vi "Save-Recall Data.vi"(0 "VISA resource name":refnum<visa-resource-name>, 1 "data type (0 : raw data)":u16(ring) items=["raw data", "error-corrected data", "error-corrected trace memory", "formatted data", "formatted memory", "formatted data / memory", "formatted data - memory"], 3 "format (0:format 1)":u16(ring) items=["format 1 (6 byte internal)", "format 2 (8 byte IEEE 32 bit float)", "format 3 (16 byte IEEE 64 bit float)", "format 4 (50 byte ASCII)"], 4 "file name (read description)":path, 5 "error in (no error)":errorcluster, 6 "save/recall":bool, 7 "saver's name":string, 8 "saved data title":string, 9 "saved data comments":string) -> (12 "recaller's name":string, 14 "VISA resource name out":refnum<visa-resource-name>, 15 "recalled data title":string, 16 "recalled data comments":string, 17 "recalled data date":string, 18 "recalled data time":string, 19 "error out":errorcluster)   [LabVIEW 2018, in "Agilent 87XX Series.lvlib"]
doc: "This VI for the HP8753B Network Analyzer is used to save and recall data and memory traces and raw data.\n\n There are many differenent data arrays which can be read out of the instrument. If a 2-port calibration is active, the \"raw data\" consists of 4 arrays. Otherwise \"raw data\" as with the other data arrays, is just one array. Each type of data is saved into a single file. \"Raw data\" just requires a little more work to be decoded from the file and written back to the instrument. \n\n \"Trace memory\" can not be written back to the instrument as memory. It must be written back to the instrument as regular data which can then be rewritten to memory using the \"data to memory\" button or VI. This only works if the \"trace memory\" was the error-corrected memory and not the formatted memory. \n\n A few important notes...\n\n Recalling data seems to be a pretty temporary thing. For example, when data is recalled it is not overwriting the data that is already in the data arrays. The recalled data will be displayed, and it will be the data stored to memory, but changing the display causes the recalled to be lost and the old data to be displayed again.\n\n Whenever formatted data is saved, the display changes to reflect the data being saved. Example, saving \"formatted memory\" causes the display to switch to \"MEMORY\". Restoring data, switches the display to \"DATA\"."
uses:
  Agilent 87XX Series.lvlib
panel:
  # "save to file\nrecall from file"
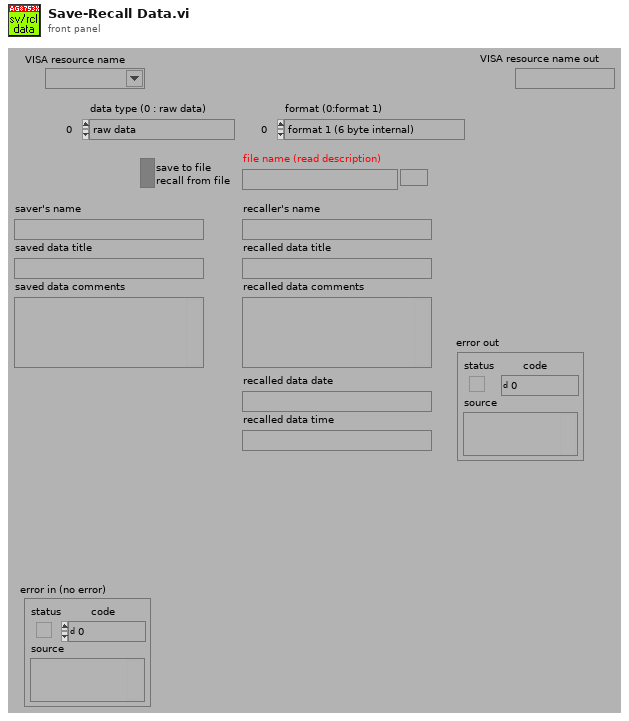
[diagram p1: front panel]
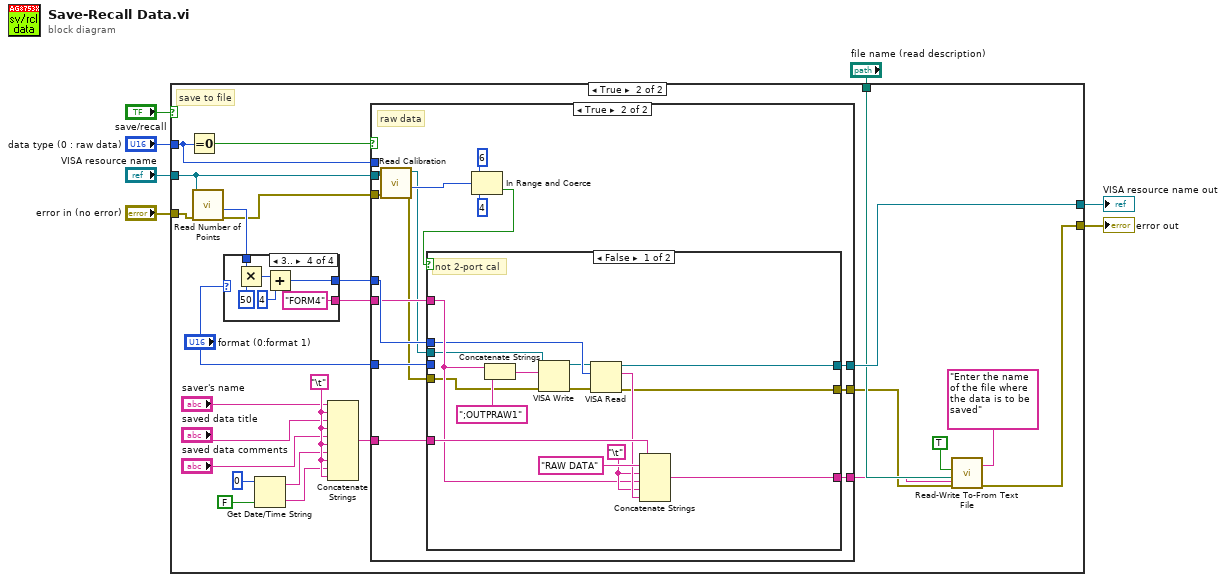
[diagram p0: block diagram]
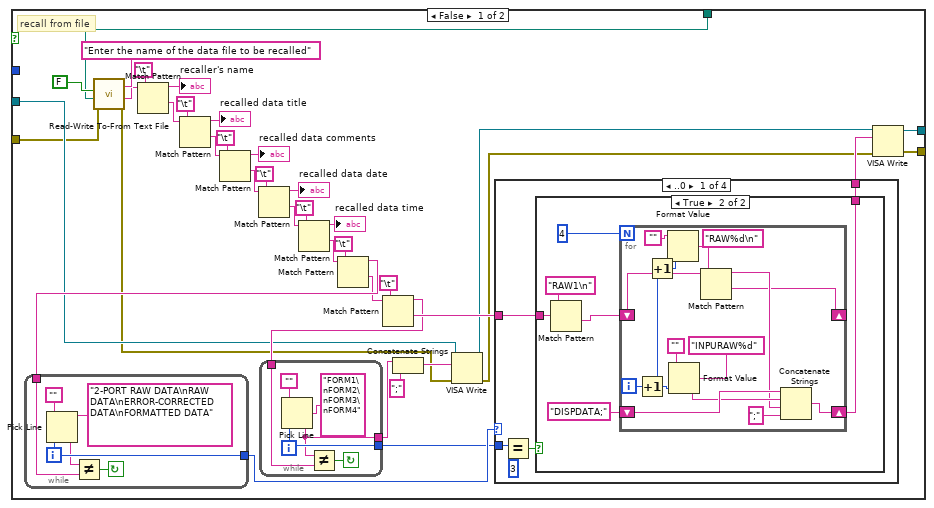
[diagram p2: hidden frame]
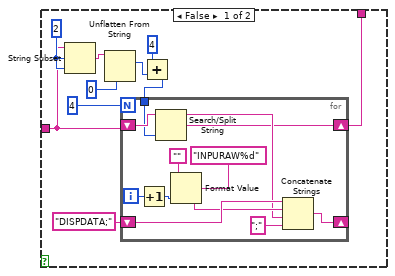
[diagram p3: hidden frame]
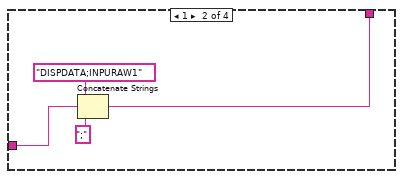
[diagram p4: hidden frame]
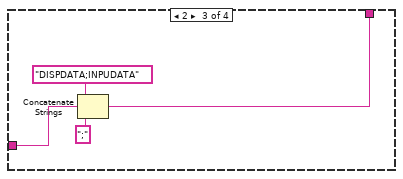
[diagram p5: hidden frame]
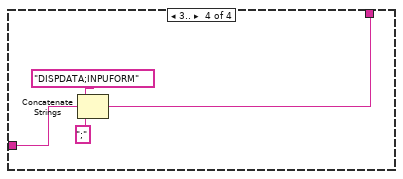
[diagram p6: hidden frame]
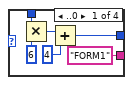
[diagram p7: hidden frame]
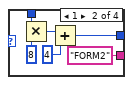
[diagram p8: hidden frame]
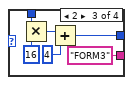
[diagram p9: hidden frame]
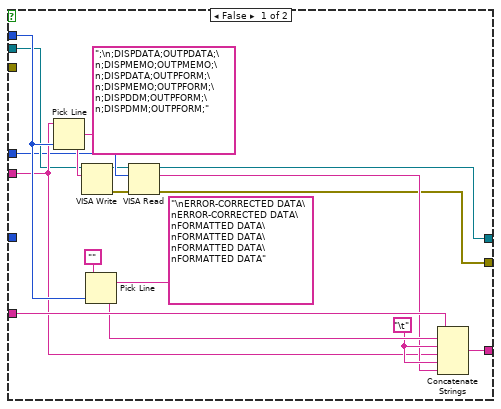
[diagram p10: hidden frame]
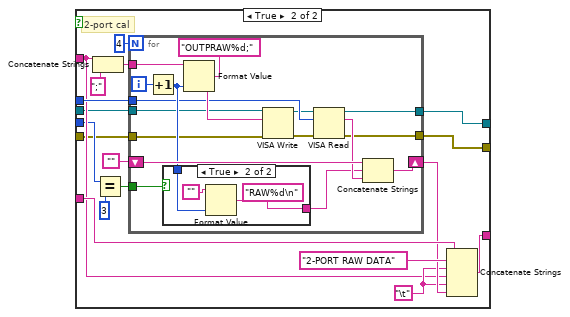
[diagram p11: hidden frame]
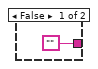
[diagram p12: hidden frame]
diagram:
  n1 = case shown="True" "save/recall" {
    tunnel: "data type (0 : raw data)" -> [_ w132]
    tunnel: "VISA resource name" -> [w18 w131]
    tunnel: "file name (read description)" -> [w12 w122]
    tunnel: "error in (no error)" -> [w9 w126]
    tunnel: [w15 w124] -> w2
    tunnel: [w14 w119] -> w1
    frame False {
      # "recall from file"
      n2 = call "Read-Write To-From Text File.vi"("dialog box prompt"="Enter the name of the data file to be recalled", "error in (no error)"=w9, "file name (read description)"=w12, "read/write (f:read)"=FALSE) -> ("error out"=w10:errorcluster, "string which was read"=w8:string)  [unwired: 6 in]
      n3 = Match Pattern(string=w8, regular expression="\t") -> (before substring=→"recaller's name":string, after substring=w42:string)  [unwired: 1 in, 2 out]
      n4 = Match Pattern(string=w42, regular expression="\t") -> (before substring=→"recalled data title":string, after substring=w41:string)  [unwired: 1 in, 2 out]
      n5 = Match Pattern(string=w41, regular expression="\t") -> (before substring=→"recalled data comments":string, after substring=w37:string)  [unwired: 1 in, 2 out]
      n6 = Match Pattern(string=w37, regular expression="\t") -> (before substring=→"recalled data date":string, after substring=w40:string)  [unwired: 1 in, 2 out]
      n7 = Match Pattern(string=w40, regular expression="\t") -> (before substring=→"recalled data time":string, after substring=w30:string)  [unwired: 1 in, 2 out]
      n8 = Match Pattern(string=w30, regular expression="\t") -> (before substring=w29:string, after substring=w27:string)  [unwired: 1 in, 2 out]
      n9 = while {
        tunnel: w29 -> [w46]
        tunnel: [w49] -> w25
        i -> [w49]
        stop <- w47 continue-if-true
        n10 = Pick Line(string ("")="", multi-line string="2-PORT RAW DATA\nRAW DATA\nERROR-CORRECTED DATA\nFORMATTED DATA", line index=w49) -> (output string=w48:string)
        n11 = Not Equal?(x=w48, y=w46) -> (x != y?=w47:bool)
      }
      n12 = Match Pattern(string=w27, regular expression="\t") -> (before substring=w24:string, after substring=w26:string)  [unwired: 1 in, 2 out]
      n13 = while {
        tunnel: [w52] -> w22
        tunnel: w24 -> [w53]
        tunnel: [w55] -> w20
        i -> [w55]
        stop <- w54 continue-if-true
        n14 = Pick Line(string ("")="", multi-line string="FORM1\nFORM2\nFORM3\nFORM4", line index=w55) -> (output string=w52:string)
        n15 = Not Equal?(x=w52, y=w53) -> (x != y?=w54:bool)
      }
      n16 = Concatenate Strings(w22, ";") -> (w21:string)
      n17 = VISA Write(VISA resource name=w18, write buffer=w21, error in (no error)=w10) -> (VISA resource name out=w17:refnum<visa-resource-name>, error out=w16:errorcluster)  [unwired: 1 out]
      n18 = case shown="..0" w25 {
        tunnel: w26 -> [w59 w108 w112 w116]
        tunnel: [w58 w106 w110 w114] -> w19
        tunnel: w20 -> [w61 _ _ _]
        frame ..0 {
          n19 = Equal?(x=w61, y=3) -> (x = y?=w60:bool)
          n20 = case shown="True" w60 {
            tunnel: w59 -> [w64 w88]
            tunnel: [w63 w85] -> w58
            frame False {
              w72 = 2
              n21 = String Subset(string=w64, offset (0)=w72, length (rest)=w72) -> (substring=w71:string)
              n22 = Unflatten From String(type=u16 0, binary string=w71) -> (value=w65:u16)  [unwired: 3 in, 2 out]
              n23 = Add(x=4, y=w65) -> (x+y=w67:i32)
              n24 = for {
                N: 4 -> [_]
                shift-right: [w73] -> w63
                shift-left: w64 -> [w84]
                tunnel: w67 -> [w83]
                shift-right: [w74] -> _
                shift-left: "DISPDATA;" -> [w78]
                i -> [w81]
                n25 = Increment(x=w81) -> (x+1=w82:i32)
                n26 = Search/Split String(string=w84, offset (0)=w83) -> (substring before match=w76:string, match + rest of string=w73:string)  [unwired: 1 in, 1 out]
                n27 = Format Value(string ("")="", format string="INPURAW%d", value (0)=w82) -> (output string=w77:string)
                n28 = Concatenate Strings(w78, w77, w76, ";") -> (w74:string)
              }
            }
            frame True {
              n29 = Match Pattern(string=w88, regular expression="RAW1\n") -> (after substring=w86:string)  [unwired: 1 in, 3 out]
              n30 = for {
                N: 4 -> [_]
                shift-right: [w91] -> _
                shift-left: w86 -> [w95]
                shift-right: [w99] -> w85
                shift-left: "DISPDATA;" -> [w102]
                i -> [w105]
                n31 = Increment(x=w105) -> (x+1=w94:i32)
                n32 = Increment(x=w94) -> (x+1=w93:i32)
                n33 = Format Value(string ("")="", format string="RAW%d\n", value (0)=w93) -> (output string=w96:string)
                n34 = Format Value(string ("")="", format string="INPURAW%d", value (0)=w94) -> (output string=w101:string)
                n35 = Match Pattern(string=w95, regular expression=w96) -> (before substring=w92:string, after substring=w91:string)  [unwired: 1 in, 2 out]
                n36 = Concatenate Strings(w102, w101, w92, ";") -> (w99:string)
              }
            }
          }
        }
        frame 1 {
          n37 = Concatenate Strings("DISPDATA;INPURAW1", w108, ";") -> (w106:string)
        }
        frame 2 {
          n38 = Concatenate Strings("DISPDATA;INPUDATA", w112, ";") -> (w110:string)
        }
        frame 3.. {
          n39 = Concatenate Strings("DISPDATA;INPUFORM", w116, ";") -> (w114:string)
        }
      }
      n40 = VISA Write(VISA resource name=w17, write buffer=w19, error in (no error)=w16) -> (VISA resource name out=w15:refnum<visa-resource-name>, error out=w14:errorcluster)  [unwired: 1 out]
    }
    frame True {
      w141 = "\t"
      # "save to file"
      n41 = Equal To 0?(x=w132) -> (x = 0?=w142:bool)
      n42 = call "Read Number of Points.vi"("error in (no error)"=w126, "VISA resource name"=w131) -> ("error out"=w125:errorcluster, "num points"=w127:i32)  [unwired: 7 in, 1 out]
      n43 = case shown="3.." "format (0:format 1)" {
        tunnel: w127 -> [w148 w154 w160 w166]
        tunnel: [w144 w150 w156 w162] -> w129
        tunnel: ["FORM1" "FORM2" "FORM3" "FORM4"] -> w128
        frame ..0 {
          n44 = Multiply(x=w148, y=6) -> (x*y=w146:i32)
          n45 = Add(x=w146, y=4) -> (x+y=w144:i32)
        }
        frame 1 {
          n46 = Multiply(x=w154, y=8) -> (x*y=w152:i32)
          n47 = Add(x=w152, y=4) -> (x+y=w150:i32)
        }
        frame 2 {
          n48 = Multiply(x=w160, y=16) -> (x*y=w158:i32)
          n49 = Add(x=w158, y=4) -> (x+y=w156:i32)
        }
        frame 3.. {
          n50 = Multiply(x=w166, y=50) -> (x*y=w164:i32)
          n51 = Add(x=w164, y=4) -> (x+y=w162:i32)
        }
      }
      n52 = Get Date/Time String(date format (0)=0, want seconds? (F)=FALSE) -> (date string=w139:string, time string=w140:string)  [unwired: 1 in]
      n53 = Concatenate Strings("saver's name", w141, "saved data title", w141, "saved data comments", w141, w139, w141, w140, w141) -> (w133:string)
      n54 = case shown="True" w142 {
        tunnel: w131 -> [w172 w190]
        tunnel: w133 -> [w178 w198]
        tunnel: [w179 w197] -> w118
        tunnel: w132 -> [w180 _]
        tunnel: w129 -> [w168 w193]
        tunnel: w128 -> [w173 w192]
        tunnel: "format (0:format 1)" -> [_ w191]
        tunnel: w125 -> [_ w188]
        tunnel: [w170 w185] -> w124
        tunnel: [w169 w184] -> w121
        frame False {
          w175 = "\t"
          n55 = Pick Line(string ("")=w173, multi-line string=";\n;DISPDATA;OUTPDATA;\n;DISPMEMO;OUTPMEMO;\n;DISPDATA;OUTPFORM;\n;DISPMEMO;OUTPFORM;\n;DISPDDM;OUTPFORM;\n;DISPDMM;OUTPFORM;", line index=w180) -> (output string=w182:string)
          n56 = VISA Write(VISA resource name=w172, write buffer=w182) -> (VISA resource name out=w167:refnum<visa-resource-name>, error out=w171:errorcluster)  [unwired: 1 in, 1 out]
          n57 = Pick Line(string ("")="", multi-line string="\nERROR-CORRECTED DATA\nERROR-CORRECTED DATA\nFORMATTED DATA\nFORMATTED DATA\nFORMATTED DATA\nFORMATTED DATA", line index=w180) -> (output string=w177:string)
          n58 = VISA Read(VISA resource name=w167, byte count=w168, error in (no error)=w171) -> (VISA resource name out=w170:refnum<visa-resource-name>, read buffer=w174:string, error out=w169:errorcluster)  [unwired: 1 out]
          n59 = Concatenate Strings(w178, w177, w175, w173, w175, w174) -> (w179:string)
        }
        frame True {
          # "raw data"
          n60 = call "Read Calibration.vi"("error in (no error)"=w188, "VISA resource name"=w190) -> ("error out"=w187:errorcluster, "cal type"=w189:i32, "VISA resource name out"=w186:refnum<visa-resource-name>)  [unwired: 7 in]
          n61 = In Range and Coerce(upper limit=6, x=w189, lower limit=4) -> (In Range?=w194:bool)  [unwired: 1 out]
          n62 = case shown="False" w194 {
            tunnel: w198 -> [w213 w229]
            tunnel: [w211 w228] -> w197
            tunnel: w193 -> [w200 w227]
            tunnel: w192 -> [w206 w222]
            tunnel: w191 -> [_ w219]
            tunnel: [w204 w217] -> w185
            tunnel: [w203 w216] -> w184
            tunnel: w187 -> [w202 w214]
            tunnel: w186 -> [w201 w215]
            frame False {
              w207 = "\t"
              # "not 2-port cal"
              n63 = Concatenate Strings(w206, ";OUTPRAW1") -> (w209:string)
              n64 = VISA Write(VISA resource name=w201, write buffer=w209, error in (no error)=w202) -> (VISA resource name out=w199:refnum<visa-resource-name>, error out=w205:errorcluster)  [unwired: 1 out]
              n65 = VISA Read(VISA resource name=w199, byte count=w200, error in (no error)=w205) -> (VISA resource name out=w204:refnum<visa-resource-name>, read buffer=w208:string, error out=w203:errorcluster)  [unwired: 1 out]
              n66 = Concatenate Strings(w213, "RAW DATA", w207, w206, w207, w208) -> (w211:string)
            }
            frame True {
              w225 = "\t"
              # "2-port cal"
              n67 = Concatenate Strings(w222, ";") -> (w221:string)
              n68 = Equal?(x=w219, y=u16 3) -> (x = y?=w218:bool)
              n69 = for {
                N: 4 -> [_]
                shift-right: [w244] -> w226
                shift-left: "" -> [w245]
                tunnel: w227 -> [w233]
                tunnel: w221 -> [w243]
                tunnel: w218 -> [w241]
                tunnel: w215 -> [w237]
                tunnel: w214 -> [w236]
                tunnel: [w235] -> w217
                tunnel: [w234] -> w216
                i -> [w248]
                n70 = Increment(x=w248) -> (x+1=w240:i32)
                n71 = case shown="True" w241 {
                  tunnel: w240 -> [_ w251]
                  tunnel: ["" w250] -> w239
                  frame False {
                  }
                  frame True {
                    n72 = Format Value(string ("")="", format string="RAW%d\n", value (0)=w251) -> (output string=w250:string)
                  }
                }
                n73 = Format Value(string ("")=w243, format string="OUTPRAW%d;", value (0)=w240) -> (output string=w246:string)
                n74 = VISA Write(VISA resource name=w237, write buffer=w246, error in (no error)=w236) -> (VISA resource name out=w232:refnum<visa-resource-name>, error out=w238:errorcluster)  [unwired: 1 out]
                n75 = VISA Read(VISA resource name=w232, byte count=w233, error in (no error)=w238) -> (VISA resource name out=w235:refnum<visa-resource-name>, read buffer=w242:string, error out=w234:errorcluster)  [unwired: 1 out]
                n76 = Concatenate Strings(w245, w239, w242) -> (w244:string)
              }
              n77 = Concatenate Strings(w229, "2-PORT RAW DATA", w225, w222, w225, w226) -> (w228:string)
            }
          }
        }
      }
      n78 = call "Read-Write To-From Text File.vi"("string to be written"=w118, "dialog box prompt"="Enter the name of the file where the data is to be saved", "error in (no error)"=w121, "file name (read description)"=w122, "read/write (f:read)"=TRUE) -> ("error out"=w119:errorcluster)  [unwired: 5 in, 1 out]
    }
  }
  "error out" <- w1
  "VISA resource name out" <- w2
